vi "String to Complex Number (CDB 1D Array).vi"(2 "use system decimal point (T)":bool=TRUE, 3 "default (0 CDB)":cdb, 4 "offset":i32, 5 "strings[]":string[](array[string])) -> (0 "numbers[]":cdb[](array[numeric]), 1 "offsets past number[]":i32[](array[numeric]))   [LabVIEW 2018, in "Numeric Data Type.lvclass"]
doc: "<b> </b> <b> </b>\n©2013, Q Software Innovations, LLC.\n\nWritten in National Instruments LabVIEW™ 2013.\n\nAuthored by Quentin Alldredge\nQ@qsoftwareinnovations.com\nwww.qsoftwareinnovations.com\n\nAll rights reserved."
uses:
  Numeric Data Type.lvclass
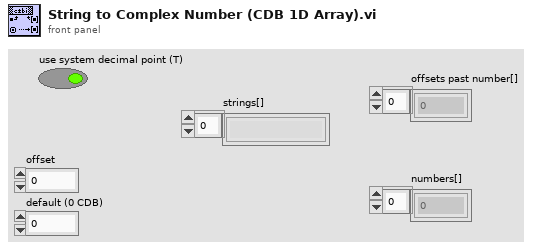
[diagram p1: front panel]
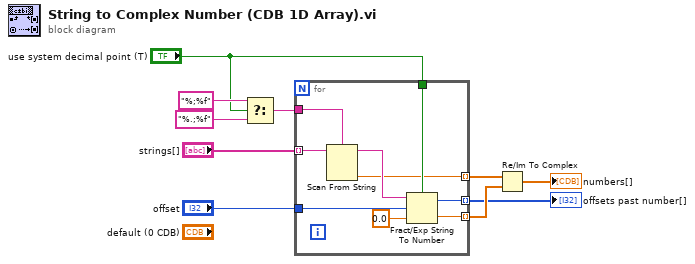
[diagram p0: block diagram]
diagram:
  n1 = Select(t="%;%f", s="use system decimal point (T)", f="%.;%f") -> (s? t:f=w8:string)
  n2 = for {
    tunnel: w8 -> [w19]
    tunnel: "use system decimal point (T)" -> [w17]
    tunnel: [w16] -> w6 mode=indexing
    tunnel: [w15] -> w5 mode=indexing
    tunnel: "offset" -> [w13]
    tunnel: [w12] -> w1 mode=indexing
    tunnel: "strings[]" -> [w11] mode=indexing
    n3 = Scan From String(format string=w19, input string=w11) -> (remaining string=w18:string, output 1=w16:dbl)  [unwired: 3 in, 2 out]
    n4 = Fract/Exp String To Number(use system decimal point (T)=w17, string=w18, offset=w13, default (0 dbl)=0.0 ("default (0 DBL)")) -> (offset past number=w12:i32, number=w15:dbl)
  }
  "offsets past number[]" <- w1
  n5 = Re/Im To Complex(1:w5, 2:w6) -> (0:→"numbers[]":cdb[])
